vi "Dropdown - Program Close.vi"(11 "Error In":errorcluster) -> (15 "Error Out":errorcluster)   [LabVIEW 2019]
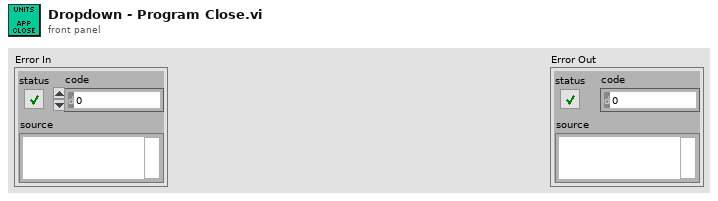
[diagram p1: front panel]
types:
  T1 = enum16{"Idle", "Reveal Dropdown", "Hide FP", "Set Options", "Close Program"}
  T2 = enum16{"Set Abbreviations", "Set Engine Mode", "Set Enum Position", "Get Abbreviation", "Write Abbreviation", "Read Enum Position", "Read Engine Mode", "Read Abbreviations", "Engine Started", "Check Engine", "Init Global", "Set Cursor", "Read Cursor"}
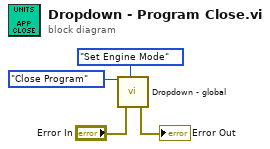
[diagram p0: block diagram]
diagram:
  n1 = call "Dropdown - global.vi"("Engine Mode In"=T1."Close Program" ("Engine Mode INN"), "Error In"="Error In", "Global Mode"=T2."Set Engine Mode") -> ("Error Out"=→"Error Out":errorcluster)  [unwired: 8 in, 8 out]
